vi "Periodic Flush Queue.vi"(8 "error in":errorcluster, 11 "Report Generator in":refnum<class "Report Generator.lvclass">) -> (0 "error out":errorcluster, 3 "Report Generator out":refnum<class "Report Generator.lvclass">)   [LabVIEW 2023, in "Report Generator.lvlib" / "Report Generator.lvclass"]
uses:
  Library/Report Generator.lvclass
  C:/Users/Public/Documents/Development/builds/Engine/Engine.lvlibp/Project/Engine.lvclass
  builds/Engine/Engine.lvlibp/Accessors/Read Report Queue.vi
  builds/Tools/QDMH.lvlibp/QDMH.lvclass
  builds/Engine/Engine.lvlibp/Project/Engine.lvclass
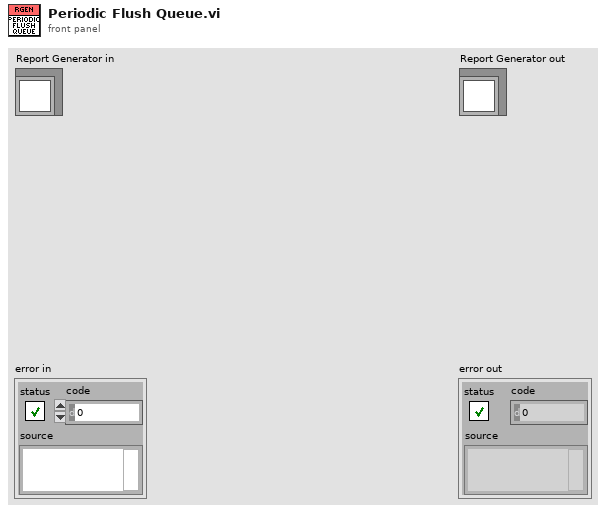
[diagram p1: front panel]
types:
  T1 = typedef "QDMH.lvlibp/QDMH.lvclass/QDMH Message.ctl" = cluster{"State":string, "Data":variant}
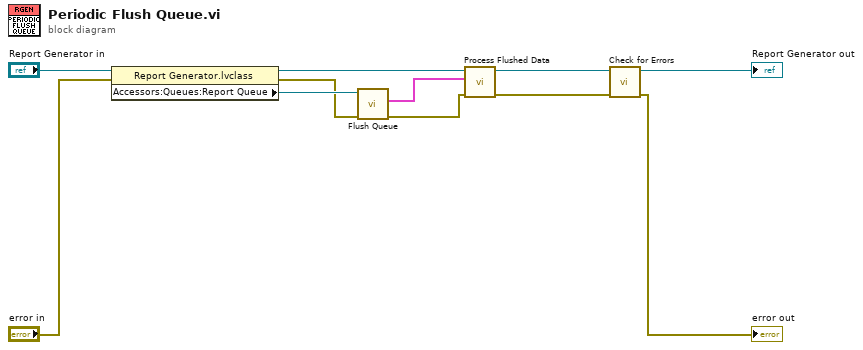
[diagram p0: block diagram]
diagram:
  n1 = property class="Report Generator.lvclass"(reference="Report Generator in", error in="error in") -> (reference out=w4:refnum<class "Report Generator.lvclass">, error out=w8:errorcluster, "Accessors:Queues:Report Queue"=w9:refnum<class "QDMH.lvclass">)
  n2 = call "Flush Queue.vi"("error in"=w8, "QDMH in"=w9) -> ("error out"=w2:errorcluster, "Flushed elements"=w5:T1[])  [unwired: 7 in, 1 out]
  n3 = call "Process Flushed Data.vi"("error in"=w2, "Flushed elements"=w5, "Report Generator in"=w4) -> ("error out"=w1:errorcluster, "Report Generator out"=w3:refnum<class "Report Generator.lvclass">)  [unwired: 7 in]
  n4 = call "Check for Errors.vi"("error in"=w1, "Engine in"=w3) -> ("error out"=→"error out":errorcluster, "Engine out"=→"Report Generator out":refnum<class "Report Generator.lvclass">)  [unwired: 8 in]
